vi "Project_2(Main).vi"() -> ()   [LabVIEW 2023]
doc: "Project 2: Finite sate machine for loading and launching passengers in the Salvia Express"
uses:
  controls/enum defining states.ctl
  controls/Boolean output indicator.ctl
  controls/Boolean L E indictaor.ctl
panel:
  out "L       E \nIndicator":T1 caption="L      E"
  out "Output\nIndicator":T2 caption="Z     Y     X"
  out "Reset?":bool
  out "Present State":T3
  in  "Stop Button":bool
  # "Salvia Express Passenger Control"
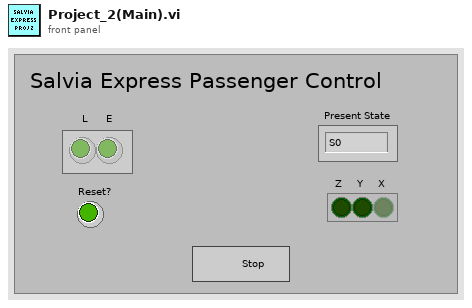
[diagram p1: front panel]
types:
  T1 = typedef "Boolean L E indictaor.ctl" = bool[]
  T2 = typedef "Boolean output indicator.ctl" = bool[]
  T3 = typedef "enum defining states.ctl" = enum16{"S0", "S1", "S2", "S3"}
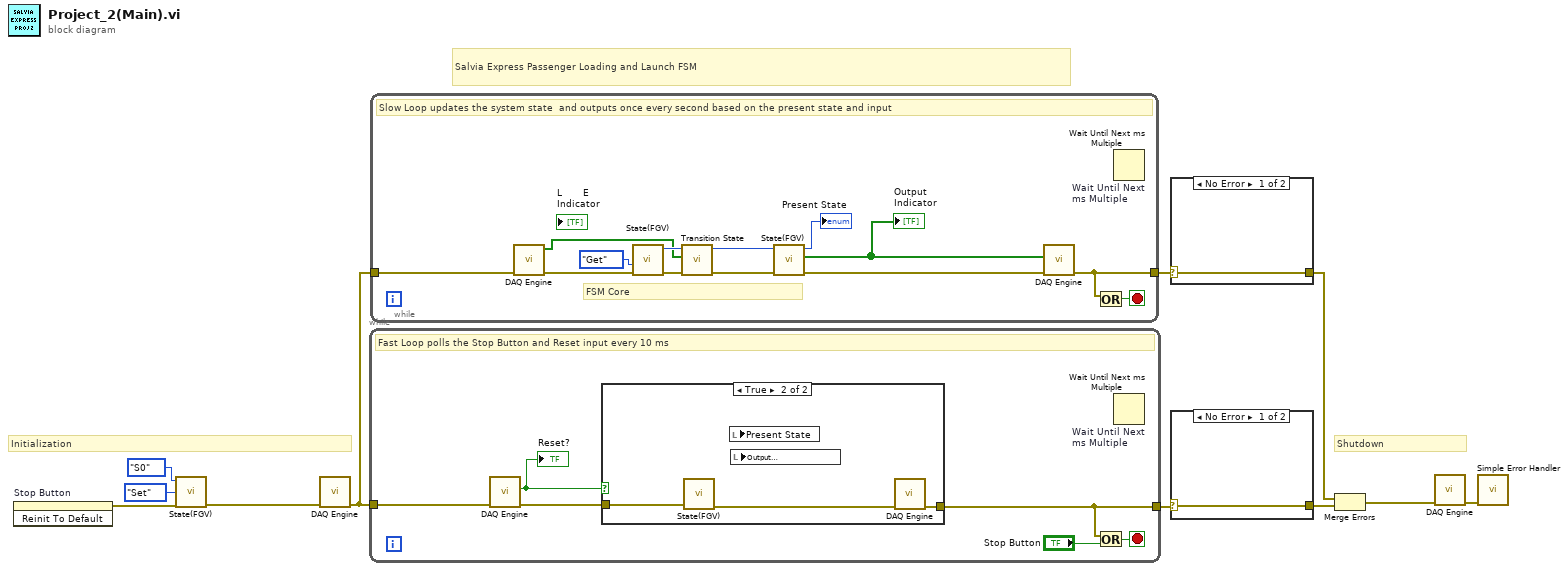
[diagram p0: block diagram]
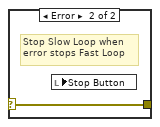
[diagram p2: hidden frame]
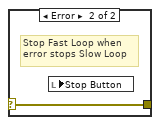
[diagram p3: hidden frame]
diagram:
  # "Shutdown"
  # "Initialization"
  # "Salvia Express Passenger Loading and Launch FSM"
  n1 = invoke on="Stop Button" class="Bool (strict)" method="Reinit To Default"() -> (error out=w6:errorcluster)  [unwired: 3 in, 2 out]
  n2 = call "State(FGV).vi"("Error In"=w6, "Action"=enum16{"Set", "Get"}."Set", "input state"=enum_defining_states."S0" ("Input State")) -> ("Error Out"=w1:errorcluster)  [unwired: 6 in, 2 out]
  n3 = call "DAQ Engine.vi"("Error In"=w1) -> ("Error Out"=w8:errorcluster)  [unwired: 8 in, 2 out]
  n4 = while {
    tunnel: w8 -> [w17]
    tunnel: [w13] -> w4
    stop <- w15 stop-if-true
    # "Fast Loop polls the Stop Button and Reset input every 10 ms"
    n5 = call "DAQ Engine.vi"("Error In"=w17) -> ("Error Out"=w16:errorcluster, "Reset ?"=w12:bool)  [unwired: 8 in, 1 out]
    "Reset?" <- w12
    n6 = case shown="True" w12 {
      tunnel: w16 -> [w18 w21]
      tunnel: [w18 w19] -> w13
      frame False {
      }
      frame True {
        n7 = call "State(FGV).vi"("Error In"=w21) -> ("Error Out"=w20:errorcluster)  [unwired: 8 in, 2 out]
        n8 = local read "Present State"() -> ()  [unwired: 1 in]
        n9 = local read "Output\nIndicator"() -> ()  [unwired: 1 in]
        n10 = call "DAQ Engine.vi"("Error In"=w20) -> ("Error Out"=w19:errorcluster)  [unwired: 8 in, 2 out]
      }
    }
    n11 = Or(x=w13, y="Stop Button") -> (x .or. y?=w15:bool)
    n12 = Wait Until Next ms Multiple "Wait Until Next \nms Multiple"() -> ()  [unwired: 1 in, 1 out]
  }
  n13 = while {
    tunnel: w8 -> [w34]
    tunnel: [w26] -> w5
    stop <- w30 stop-if-true
    # "FSM Core"
    # "Slow Loop updates the system state  and outputs once every second based on the present state and input"
    n14 = call "DAQ Engine.vi"("Error In"=w34) -> ("Error Out"=w25:errorcluster, "L       E \nIndicator"=w24:T1)  [unwired: 8 in, 1 out]
    n15 = call "State(FGV).vi"("Error In"=w25, "Action"=enum16{"Set", "Get"}."Get") -> ("Error Out"=w32:errorcluster, "output state"=w31:T3)  [unwired: 7 in, 1 out]
    n16 = call "Transition State.vi"("Error In"=w32, "L       E \nIndicator"=w24, "Present  State"=w31) -> ("Error Out"=w28:errorcluster, "Next State"=w29:T3)  [unwired: 7 in]
    n17 = call "State(FGV).vi"("Error In"=w28, "input state"=w29) -> ("Error Out"=w27:errorcluster, "Output \nIndicator"=w22:T2, "output state"=→"Present State":T3)  [unwired: 7 in]
    "Output\nIndicator" <- w22
    n18 = call "DAQ Engine.vi"("Error In"=w27, "Output \nIndicator"=w22) -> ("Error Out"=w26:errorcluster)  [unwired: 7 in, 2 out]
    n19 = Or(x=w26) -> (x .or. y?=w30:bool)  [unwired: 1 in]
    n20 = Wait Until Next ms Multiple "Wait Until Next \nms Multiple"() -> ()  [unwired: 1 in, 1 out]
  }
  n21 = case shown="No Error" w5 {
    selector: w5 -> [w35 w36]
    tunnel: [w35 w36] -> w2
    frame No Error {
    }
    frame Error {
      # "Stop Fast Loop when\nerror stops Slow Loop"
      n22 = local read "Stop Button"() -> ()  [unwired: 1 in]
    }
  }
  n23 = case shown="No Error" w4 {
    selector: w4 -> [w37 w38]
    tunnel: [w37 w38] -> w3
    frame No Error {
    }
    frame Error {
      # "Stop Slow Loop when\nerror stops Fast Loop"
      n24 = local read "Stop Button"() -> ()  [unwired: 1 in]
    }
  }
  n25 = Merge Errors(w2, w3) -> (w7:errorcluster)
  n26 = call "DAQ Engine.vi"("Error In"=w7) -> ("Error Out"=w9:errorcluster)  [unwired: 8 in, 2 out]
  n27 = call <vilib>:"Simple Error Handler.vi"("error in (no error)"=w9) -> ()  [unwired: 4 in, 5 out]
